vi "Code128Build-Zxing.vi"(2 "ScaleY":u8=4, 3 "ScaleX":u8=1, 5 "Text":string="ZY201801") -> (1 "out Array":bool[][](array[boolean]))   [LabVIEW 2018]
uses:
  zxing.dll
  System.Drawing
panel:
  out "大小":i32[](array[numeric])
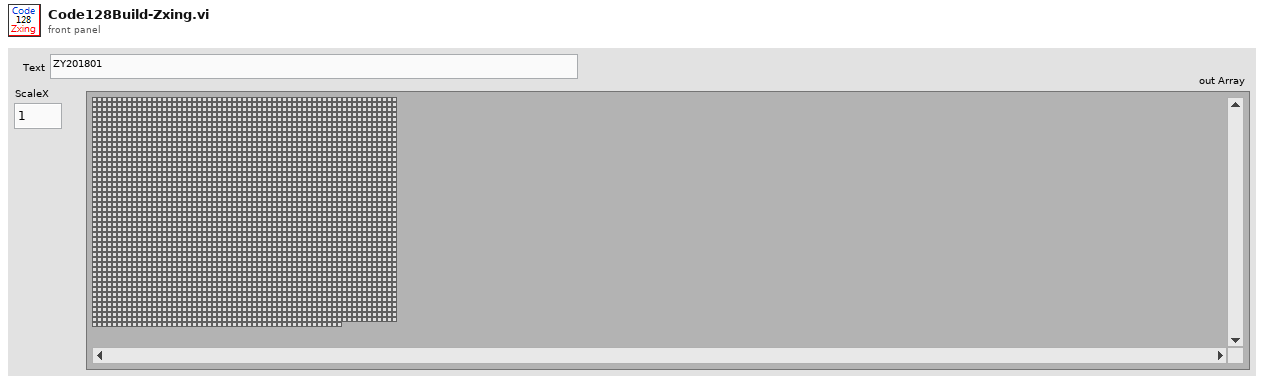
[diagram p1: front panel]
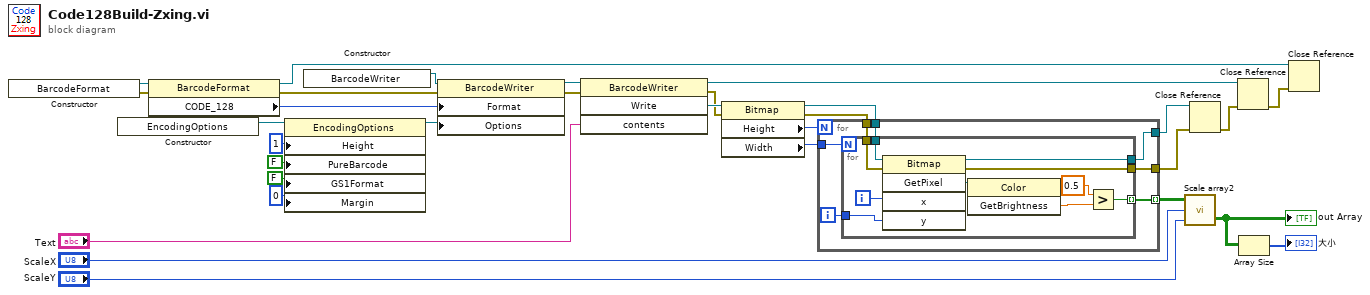
[diagram p0: block diagram]
diagram:
  n1 = constructor class="BarcodeFormat"() -> (reference out=w13:refnum<k24>, error out=w31:errorcluster)  [unwired: 3 in, 1 out]
  n2 = constructor class="EncodingOptions"() -> (reference out=w10:refnum<k24>)  [unwired: 3 in, 2 out]
  n3 = property class="BarcodeFormat"(reference=w13, error in=w31) -> (reference out=w14:refnum<k24>, error out=w21:errorcluster, "CODE_128"=w1:i32)
  n4 = property class="EncodingOptions"(reference=w10, "Height"=1, "PureBarcode"=FALSE, "GS1Format"=FALSE, "Margin"=0) -> (reference out=w12:refnum<k24>)  [unwired: 1 in, 1 out]
  n5 = constructor class="BarcodeWriter"() -> (reference out=w27:refnum<k24>)  [unwired: 3 in, 2 out]
  n6 = property class="BarcodeWriter"(reference=w27, error in=w21, "Format"=w1, "Options"=w12) -> (reference out=w29:refnum<k24>, error out=w30:errorcluster)
  n7 = invoke class="BarcodeWriter" method="Write"(reference=w29, error in=w30, "contents"="Text") -> (reference out=w23:refnum<k24>, error out=w20:errorcluster, "Write"=w24:refnum<k24>)  [unwired: 1 in, 1 out]
  n8 = property class="Bitmap"(reference=w24, error in=w20) -> (reference out=w19:refnum<k24>, error out=w18:errorcluster, "Height"=w26:i32, "Width"=w25:i32)
  n9 = for {
    N: w26 -> [_]
    tunnel: w25 -> [w38]
    tunnel: [w36] -> w9 mode=indexing
    tunnel: [w35] -> w16
    tunnel: [w34] -> w17
    tunnel: w19 -> [w33]
    tunnel: w18 -> [w32]
    i -> [w37]
    n10 = for {
      N: w38 -> [_]
      tunnel: w37 -> [w47]
      tunnel: [w41] -> w36 mode=indexing
      tunnel: [w46] -> w35
      tunnel: [w45] -> w34
      tunnel: w33 -> [w44]
      tunnel: w32 -> [w43]
      i -> [w48]
      n11 = invoke class="Bitmap" method="GetPixel"(reference=w44, error in=w43, "x"=w48, "y"=w47) -> (reference out=w46:refnum<k24>, error out=w45:errorcluster, "GetPixel"=w42:refnum<k24>)  [unwired: 1 in, 2 out]
      n12 = invoke class="Color" method="GetBrightness"(reference=w42) -> ("GetBrightness"=w39:sgl)  [unwired: 2 in, 2 out]
      n13 = Greater?(x=sgl 0.5 ("y"), y=w39) -> (0:w41:bool)
    }
  }
  n14 = call "Scale array2.vi"("ScaleY"="ScaleY", "ScaleX"="ScaleX", "in Array"=w9) -> ("out Array"=w3:bool[][])  [unwired: 2 in]
  "out Array" <- w3
  n15 = Close Reference(reference=w16, error in (no error)=w17) -> (error out=w22:errorcluster)
  n16 = Close Reference(reference=w23, error in (no error)=w22) -> (error out=w15:errorcluster)
  n17 = Array Size(array=w3) -> (size(s)=→"大小":i32[])
  n18 = Close Reference(reference=w14, error in (no error)=w15) -> ()  [unwired: 1 out]
